vi "Get DBClicked Tag Object.vi"(8 "error in (no error)":errorcluster caption="错误输入（无错误）", 11 "Tree Class 输入":refnum<class "Tree Class.lvclass"> caption="DNL_LabVIEW Object in") -> (0 "error out":errorcluster caption="错误输出", 2 "Tag":refnum<class "Tree Tag Class.lvclass">, 3 "Tree Class 输出":refnum<class "Tree Class.lvclass"> caption="DNL_LabVIEW Object out")   [LabVIEW 2012, in "Tree Tools.lvlib" / "Tree Class.lvclass"]
uses:
  Tree Class.lvclass
  Tree Tag Class/Tree Tag Class.lvclass
  Tree Class.lvclass/Tree Class.ctl
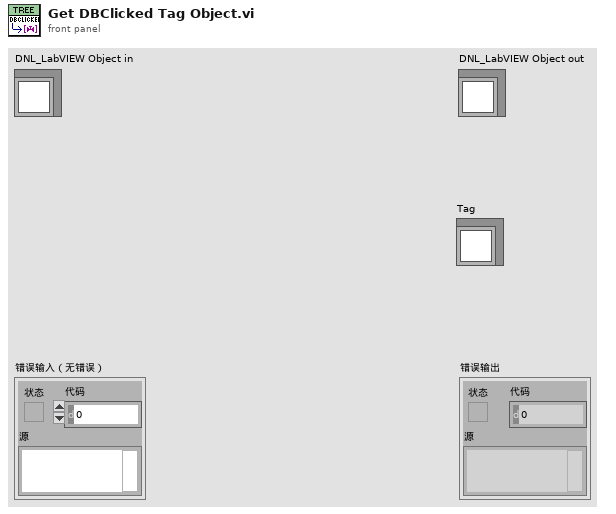
[diagram p1: front panel]
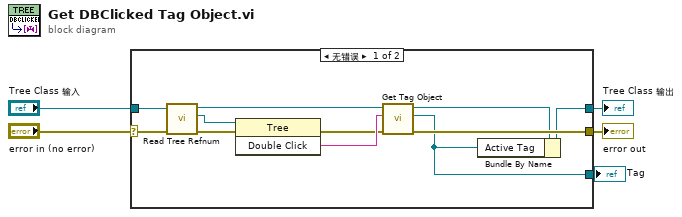
[diagram p0: block diagram]
diagram:
  n1 = case shown="无错误" "error in (no error)" {
    selector: "error in (no error)" -> [w15 w18]
    tunnel: [w9 w18] -> w4
    tunnel: [w7 w17] -> w2
    tunnel: "Tree Class 输入" -> [w16 w17]
    tunnel: [w6 _] -> w1
    frame No Error {
      n2 = call-dynamic "Read Tree Refnum.vi"("error in (no error)"=w15, "Tree_LVOOP__lava_lib_tree_class in"=w16) -> ("error out"=w11:errorcluster, "Tree Refnum"=w14:refnum<vi>, "Tree_LVOOP__lava_lib_tree_class out"=w13:refnum<class "Tree Class.lvclass">)  [unwired: 7 in]
      n3 = invoke class="Tree" method="Double Click"(reference=w14, error in=w11) -> (error out=w10:errorcluster, "Double Click"=w12:string)  [unwired: 1 in, 1 out]
      n4 = call-dynamic "Get Tag Object.vi"("error in (no error)"=w10, "Tag (string)"=w12, "Tree_LVOOP in"=w13) -> ("error out"=w9:errorcluster, "Tag"=w6:refnum<class "Tree Tag Class.lvclass">, "Tree_LVOOP out"=w8:refnum<class "Tree Class.lvclass">)  [unwired: 5 in, 1 out]
      n5 = Bundle By Name(cluster=w8, "Active Tag"=w6) -> (w7:refnum<class "Tree Class.lvclass">)
    }
    frame Error {
    }
  }
  "error out" <- w4
  "Tree Class 输出" <- w2
  "Tag" <- w1
